vi "MPB_9208 AI_0_16.vi"(10 "9208":T1) -> ()   [LabVIEW 2020]
uses:
  controls/AI_0_15.ctl
panel:
  out "Chiller Flow Rate Temp":dbl
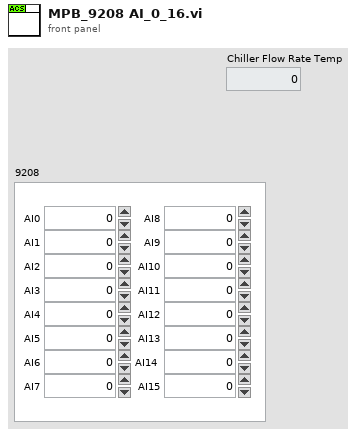
[diagram p1: front panel]
types:
  T1 = typedef "AI_0_15.ctl" = cluster{"AI0":dbl, "AI1":dbl, "AI2":dbl, "AI3":dbl, "AI4":dbl, "AI5":dbl, "AI6":dbl, "AI7":dbl, "AI8":dbl, "AI9":dbl, "AI10":dbl, "AI11":dbl, "AI12":dbl, "AI13":dbl, "AI14":dbl, "AI15":dbl}
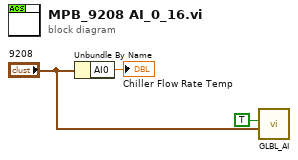
[diagram p0: block diagram]
diagram:
  n1 = Unbundle By Name("9208") -> ("AI0"=→"Chiller Flow Rate Temp":dbl)
  n2 = call "GLBL_AI.vi"("analog in 0_15"="9208", "write_read"=TRUE) -> ()  [unwired: 9 in, 1 out]
